vi "DAQ setup_trigger.vi"(0 "Vx_min":dbl, 1 "Vx_max":dbl, 2 "数组":waveform(dbl)[](array[waveform]), 5 "rate":dbl, 7 "physical channels write":tag, 9 "Timing source":tag, 11 "error in":errorcluster caption="错误输入", 12 "sample mode":enum32{"有限采样", "连续采样"}(ring), 13 "physical channels read":tag, 14 "Number of samples per channel":i32) -> (4 "Writing task out":refnum<k21>, 6 "Reading task out":refnum<k21>, 15 "错误输出":errorcluster)   [LabVIEW 2013]
uses:
  <vilib>/DAQmx/write.llb/DAQmx Write (Analog 1D Wfm NChan NSamp).vi
  <vilib>/DAQmx/create/channels.llb/DAQmx Create Channel (AO-Voltage-Basic).vi
  <vilib>/DAQmx/configure/timing.llb/DAQmx Timing (Sample Clock).vi
  <vilib>/DAQmx/create/channels.llb/DAQmx Create Channel (AI-Voltage-Basic).vi
  <vilib>/DAQmx/configure/trigger.llb/DAQmx Start Trigger (Analog Edge).vi
  <vilib>/DAQmx/miscellaneous.llb/DAQmx Fill In Error Info.vi
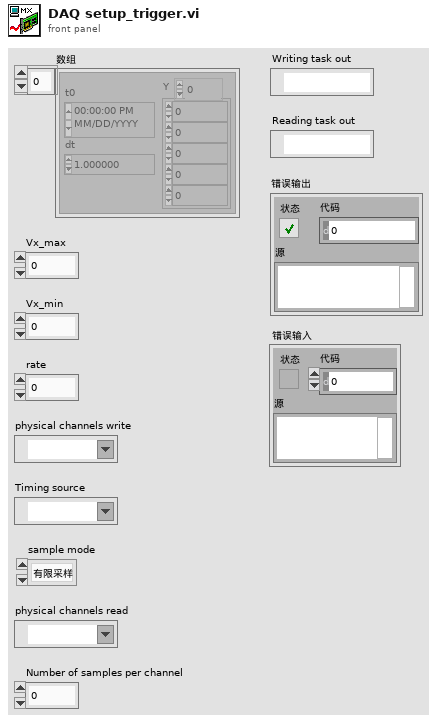
[diagram p1: front panel]
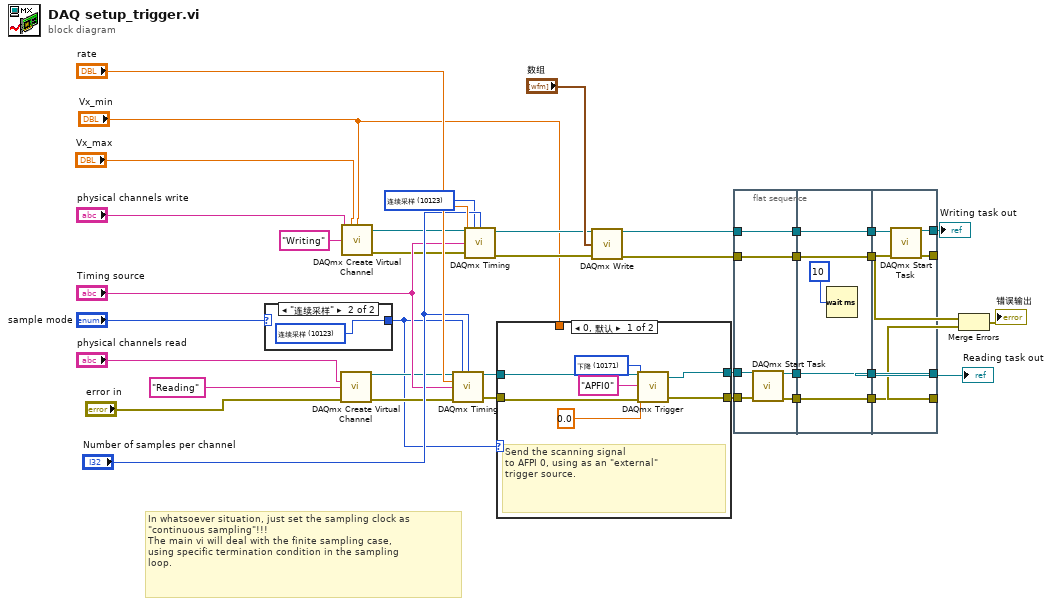
[diagram p0: block diagram]
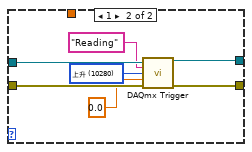
[diagram p2: hidden frame]
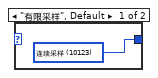
[diagram p3: hidden frame]
diagram:
  w10 = 10123 items=["有限采样"=10178, "连续采样"=10123, "硬件定时单点"=12522] ("sample mode")
  # "In whatsoever situation, just set the sampling clock as\n\"continuous sampling\"!!!\nThe main vi will deal with the finite sampling case,\nusing specific termination condition in the sampling\nloop."
  n1 = case shown="\"连续采样\"" "sample mode" {
    tunnel: [w40 w41] -> w19
    frame "有限采样", Default {
      w40 = 10123 items=["有限采样"=10178, "连续采样"=10123, "硬件定时单点"=12522] ("sample mode")
    }
    frame "连续采样" {
      w41 = 10123 items=["有限采样"=10178, "连续采样"=10123, "硬件定时单点"=12522] ("sample mode")
    }
  }
  n2 = call-poly <vilib>:"DAQmx Create Virtual Channel.vi"("physical channels"="physical channels read", "name to assign"="Reading", "error in"="error in") -> ("task out"=w22:refnum<k21>, "error out"=w23:errorcluster)  [unwired: 11 in]
  n3 = call-poly <vilib>:"DAQmx Create Virtual Channel.vi"("maximum value"="Vx_max", "minimum value"="Vx_min", "physical channels"="physical channels write", "name to assign"="Writing") -> ("task out"=w27:refnum<k21>, "error out"=w28:errorcluster)  [unwired: 10 in]
  n4 = call-poly <vilib>:"DAQmx Timing.vi"("task/channels in"=w22, "sample mode"=w19, "samples per channel"="Number of samples per channel", "rate"="rate", "source"="Timing source", "error in"=w23) -> ("task out"=w37:refnum<k21>, "error out"=w38:errorcluster)  [unwired: 8 in]
  n5 = call-poly <vilib>:"DAQmx Timing.vi"("task/channels in"=w27, "sample mode"=w10, "samples per channel"="Number of samples per channel", "rate"="rate", "source"="Timing source", "error in"=w28) -> ("task out"=w24:refnum<k21>, "error out"=w25:errorcluster)  [unwired: 8 in]
  n6 = case shown="0, 默认" w19 {
    tunnel: [w47 w55] -> w39
    tunnel: w38 -> [w45 w54]
    tunnel: w37 -> [w48 w53]
    tunnel: [w46 w49] -> w17
    tunnel: "Vx_min" -> [_ _]
    frame 0, Default {
      w44 = 10171 items=["上升"=10280, "下降"=10171] ("slope")
      # "Send the scanning signal\nto AFPI 0, using as an \"external\"\ntrigger source."
      n7 = call-poly <vilib>:"DAQmx Trigger.vi"("task/channels in"=w48, "source"="APFI0", "slope"=w44, "level"=0.0, "error in"=w45) -> ("task out"=w47:refnum<k21>, "error out"=w46:errorcluster)  [unwired: 9 in]
    }
    frame 1 {
      w51 = 10280 items=["上升"=10280, "下降"=10171] ("slope")
      n8 = call-poly <vilib>:"DAQmx Trigger.vi"("task/channels in"=w53, "source"="Reading", "slope"=w51, "level"=0.0, "error in"=w54) -> ("task out"=w55:refnum<k21>, "error out"=w49:errorcluster)  [unwired: 9 in]
    }
  }
  n9 = call-poly <vilib>:"DAQmx Write.vi"("task/channels in"=w24, "data"="数组", "error in"=w25) -> ("task out"=w16:refnum<k21>, "error out"=w14:errorcluster)  [unwired: 10 in, 1 out]
  n10 = flat-sequence {
    tunnel: w39 -> [w61]
    tunnel: w17 -> [w59]
    tunnel: [w60] -> w9
    tunnel: w16 -> [w58]
    tunnel: [w58] -> w7
    tunnel: [w57] -> w5
    tunnel: w14 -> [w57]
    tunnel: [w56] -> w3
    tunnel: w9 -> [w66]
    tunnel: [w66] -> w8
    tunnel: w7 -> [w65]
    tunnel: [w65] -> w6
    tunnel: w5 -> [w64]
    tunnel: [w64] -> w4
    tunnel: w3 -> [w63]
    tunnel: [w63] -> w2
    tunnel: [w72] -> w26
    tunnel: w8 -> [w72]
    tunnel: w6 -> [w71]
    tunnel: [w70] -> w15
    tunnel: w4 -> [w69]
    tunnel: [w68] -> w13
    tunnel: [w67] -> w12
    tunnel: w2 -> [w67]
    frame #0 {
      n11 = call <vilib>:"DAQmx Start Task.vi"("task/channels in"=w61, "error in"=w59) -> ("task out"=w60:refnum<k21>, "error out"=w56:errorcluster)  [unwired: 12 in]
    }
    frame #1 {
      n12 = Wait (ms)(milliseconds to wait=u32 10 ("等待时间（毫秒）")) -> ()  [unwired: 1 out]
    }
    frame #2 {
      n13 = call <vilib>:"DAQmx Start Task.vi"("task/channels in"=w71, "error in"=w69) -> ("task out"=w70:refnum<k21>, "error out"=w68:errorcluster)  [unwired: 12 in]
    }
  }
  n14 = Merge Errors(w13, w12) -> (→"错误输出":errorcluster)
  "Reading task out" <- w26
  "Writing task out" <- w15
